vi "Top_Level_Control_1SDI_v00.vi"() -> ()   [LabVIEW 2011]
uses:
  Strict Type Defs/Control GUI 1SDI HD.ctl
  Strict Type Defs/PII Gains.ctl
  Strict Type Defs/I16 white control.ctl
  Strict Type Defs/Thresh slider.ctl
  Strict Type Defs/Lock or Hold.ctl
  Strict Type Defs/Scan Freq Slider.ctl
  Strict Type Defs/Gains negative horizontal.ctl
  Strict Type Defs/Slider and display.ctl
  Strict Type Defs/theta 1SDI.ctl
  Strict Type Defs/Control GUI 1SDI EPR.ctl
  Strict Type Defs/Lock Select 1SDI.ctl
  Strict Type Defs/Scope and Safety.ctl
  Strict Type Defs/Hold All.ctl
  <vilib>/userdefined/High Color/nirio_resource_hc.ctl
  Strict Type Defs/Extras 1SDI.ctl
  Strict Type Defs/Double ISDI control.ctl
  Strict Type Defs/I16 1SDI Control.ctl
  <vilib>/FPGAPlugInAG/PXI-7852R/niLvFpga_Open_PXI-7852R.vi
  <vilib>/rvi/interface/common/dynamic/niFpgaDynamicAddResources.vi
  <vilib>/Utility/error.llb/Error Cluster From Error Code.vi
  <vilib>/rvi/errors/niLvFpgaAdjustHostInterfaceError.vi
  <vilib>/FPGAPlugInAG/Dynamic/niLvFpga_Close_Dynamic.vi
  <vilib>/rvi/interface/nirviOpenFPGA/nirviOpenFPGA.xnode
  FPGA Bitfiles/1SDI_FPGATarget_1SDIFPGAv00_0D511EDE.lvbitx
  <vilib>/rvi/interface/nirviReadWriteControl/nirviReadWriteControl.xnode
  <vilib>/rvi/interface/nirviMethod/nirviMethod.xnode
  <vilib>/rvi/interface/nirviCloseFPGA/nirviCloseFPGA.xnode
  <vilib>/FPGAPlugInAG/Dynamic/niLvFpga_ReadFifo_Dynamic.vi
  <vilib>/rvi/errors/niLvFpgaMergeErrorWithErrorCode.vi
  NiFpgaLv.dll
  <vilib>/rvi/interface/Simulation/niFpgaSimulationCallBeginRW.vi
panel:
  in  "watertank":bool
  out "Water Tank":dbl(slide)=-0.29411764705882354 scale=-0.3..0.3
  out "Top Loop Count":i32=272090
  in  "stop":bool
  in  "Hold All":T1
  in  "Extra Controls":enum32{"Scope", "Extra Controls", "X-Y Resurge"}(tab)
  in  "Scope+Safety":T2={"Safety First"={"lim reset"=FALSE, "no limit"=FALSE, "pos slew rate * dt"=12, "neg slew rate * dt"=-12, "Count(Ticks)"=0}, "Scope IPs"={"Trigger Direction"=enum."minus-plus", "Trigger Delay (ms)"=0.0, "Aquisition Rate (kHz)"=4000.0, "Trigger Offset (V)"=0.0, "Scale Offset"={"Scaling"={"Error signal"=1, "Output"=0, "DC Monitor"=1, "Threshold"=1}, "Offset"={"Error Signal"=0, "Output"=0, "DC Monitor"=0, "Threshold"=0}}}}
  in  "Extras 1SDI":T3={"Error Bit Shift "={"EPR BS"=0, "HD A x"=0, "HD A p"=0, "HD B x"=0, "HD B p"=0}, "I Max value"=20000, "Scan Offset"={"EPR BS"=0.0, "HD A"=0.0, "HD B"=0.0}, "Scan Ampl."={"EPR BS"=0.0, "HD A"=0.0, "HD B"=0.0}, "Scan-PII thresh"={"EPR BS"=0, "Homodyne A"=0, "Homodyne B"=0}, "Re-Scan thresh"={"EPR BS"=1000, "Homodyne A"=1000, "Homodyne B"=1000}, "Post-Offset"={"HD A x"=0.0, "HD A p"=0.0, "HD B x"=0.0, "HD B p"=0.0}}
  out "Graph error":errorcluster
  in  "Number of Elements":u32=4095
  in  "1SDI_FPGA_v00":T6="RIO1" caption="RIO Device"
  out "xy HD A":cluster{i16[], i16[]}(graph)
  in  "XY HD ON":bool
  out "xy HD B":cluster{i16[], i16[]}(graph)
  in  "Scope":T7=TRUE
  out "Scope Graph":cluster{dbl[], dbl[]}[](graph)
  in  "Lock Select":T8=enum."Homodyne B"
  in  "EPR BS":T9={"Offset Error"=-0.0003333333333333334, "Gain Error"=1, "P Gain"=25, "P Bit Shift"=-10, "I Bit Shift"=-10, "I Gain"=23, "Lock Threshold"=22, "Lock"=FALSE, "Hold"=FALSE, "Scan Frequency"=17, "Scan Bit Shift"=-4, "Gains +/- "=FALSE, "Pre- Offset Error"=0.0005084745762711861} {"Pre- Offset Error" scale=-0.01..0.01 scale format="%#_5f"; "Scan Frequency" scale=1.0..30.0; "I Gain" scale=0.0..50.0; "P Gain" scale=0.0..50.0; "Offset Error" scale=-0.01..0.01 scale format="%#_5f"}
  in  "Homodyne A":T16={"P Gain"=27, "P Bit Shift"=-8, "I Bit Shift"=-8, "I Gain"=19, "Lock Threshold"=37, "Lock"=FALSE, "Hold"=FALSE, "Scan Frequency"=13, "Scan Bit Shift"=-5, "Gains +/- "=FALSE, "Pre- Offset x"=0.0008474576271186437, "Pre-Offset p"=-0.0023163841807909607, "Gain Error x"=1, "Lock Angle"=0.0, "Gain Error p\n\n"=1} {"Lock Angle" min=-90.0 max=90.0 scale=-90.0..90.0 scale format="%#_2g"; "Pre-Offset p" scale=-0.01..0.01 scale format="%#_5f"; "Pre- Offset x" scale=-0.01..0.01 scale format="%#_5f"; "Scan Frequency" scale=1.0..30.0; "I Gain" scale=0.0..50.0; "P Gain" scale=0.0..50.0}
  in  "Homodyne B":T16={"P Gain"=14, "P Bit Shift"=-8, "I Bit Shift"=-8, "I Gain"=22, "Lock Threshold"=48, "Lock"=FALSE, "Hold"=FALSE, "Scan Frequency"=19, "Scan Bit Shift"=-5, "Gains +/- "=FALSE, "Pre- Offset x"=-0.0016384180790960455, "Pre-Offset p"=-0.002090395480225989, "Gain Error x"=1, "Lock Angle"=15.0, "Gain Error p\n\n"=1} {"Lock Angle" min=-90.0 max=90.0 scale=-90.0..90.0 scale format="%#_2g"; "Pre-Offset p" scale=-0.01..0.01 scale format="%#_5f"; "Pre- Offset x" scale=-0.01..0.01 scale format="%#_5f"; "Scan Frequency" scale=1.0..30.0; "I Gain" scale=0.0..50.0; "P Gain" scale=0.0..50.0}
  # "Error Signal"
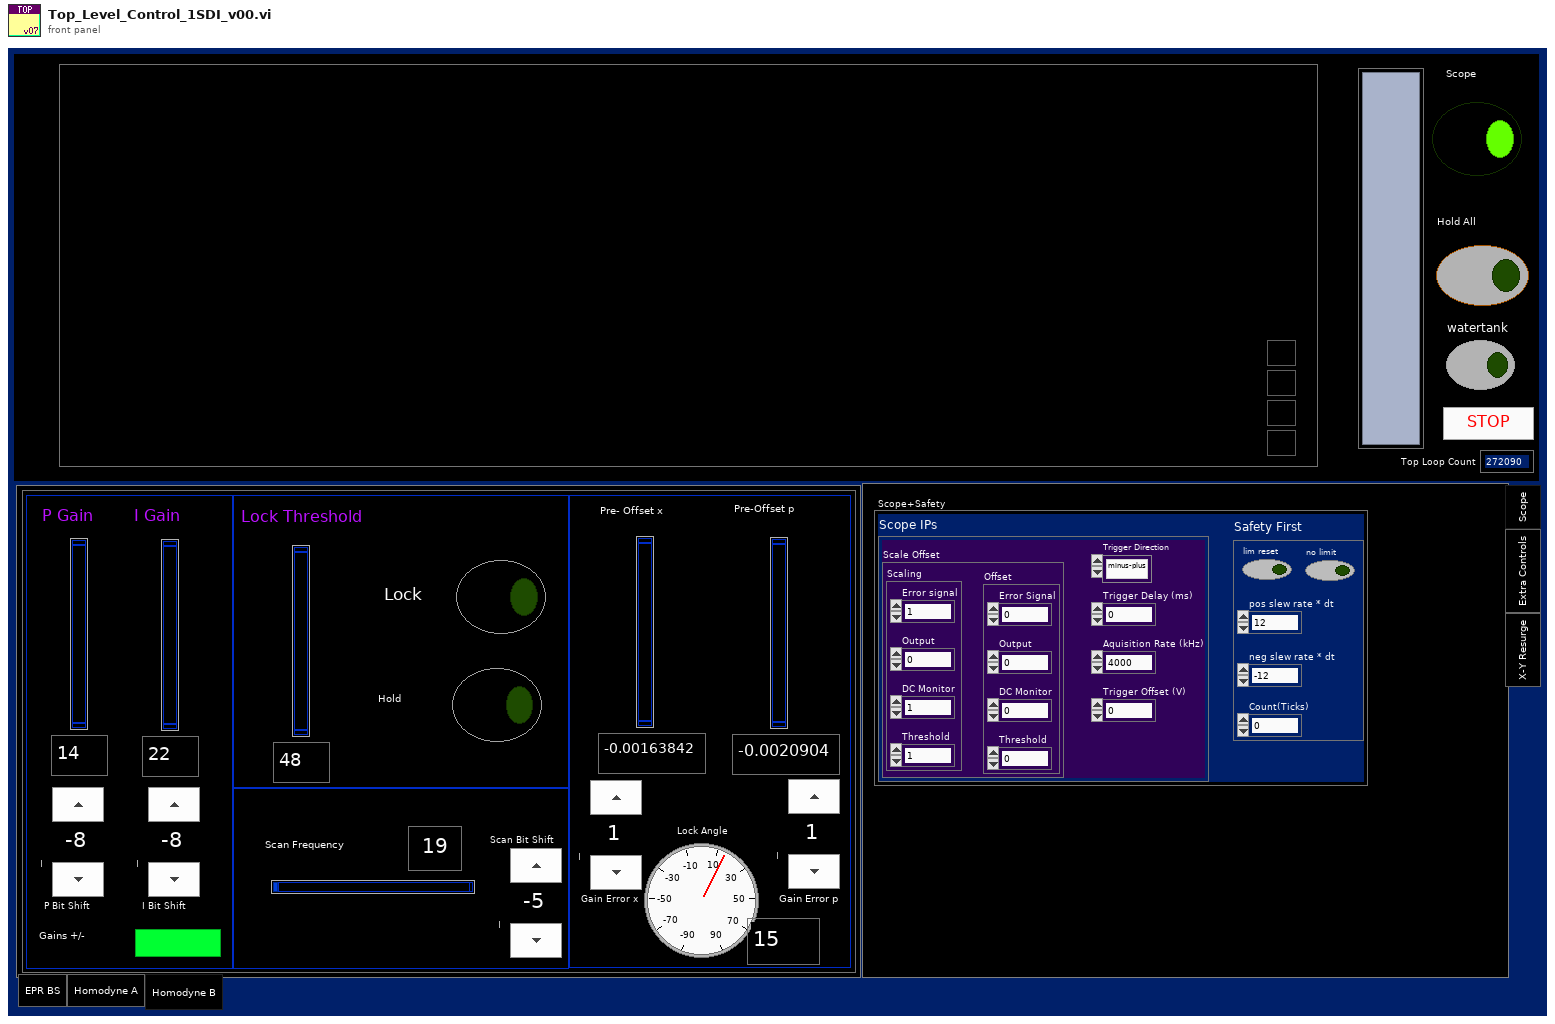
[diagram p1: front panel]
types:
  T1 = typedef "Hold All.ctl" = bool
  T2 = typedef "Scope and Safety.ctl" = cluster{"Safety First":cluster{"lim reset":bool, "no limit":bool, "pos slew rate * dt":i16, "neg slew rate * dt":i16, "Count(Ticks)":u32}, "Scope IPs":cluster{"Trigger Direction":enum8{"either", "minus-plus", "plus-minus"}, "Trigger Delay (ms)":dbl, "Aquisition Rate (kHz)":dbl, "Trigger Offset (V)":dbl, "Scale Offset":cluster{"Scaling":cluster{"Error signal":i16, "Output":i16, "DC Monitor":i16, "Threshold":i16}, "Offset":cluster{"Error Signal":i16, "Output":i16, "DC Monitor":i16, "Threshold":i16}}}}
  T3 = typedef "Extras 1SDI.ctl" = cluster{"Error Bit Shift ":cluster{"EPR BS":i16, "HD A x":i16, "HD A p":i16, "HD B x":i16, "HD B p":i16}, "I Max value":i32, "Scan Offset":T4, "Scan Ampl.":T4, "Scan-PII thresh":T5, "Re-Scan thresh":T5, "Post-Offset":cluster{"HD A x":dbl, "HD A p":dbl, "HD B x":dbl, "HD B p":dbl}}
  T4 = typedef "Double ISDI control.ctl" = cluster{"EPR BS":dbl, "HD A":dbl, "HD B":dbl}
  T5 = typedef "I16 1SDI Control.ctl" = cluster{"EPR BS":i16, "Homodyne A":i16, "Homodyne B":i16}
  T6 = typedef "nirio_resource_hc.ctl" = tag
  T7 = typedef "Lock or Hold.ctl" = bool
  T8 = typedef "Lock Select 1SDI.ctl" = enum32{"EPR BS", "Homodyne A", "Homodyne B"}
  T9 = typedef "Control GUI 1SDI EPR.ctl" = cluster{"Offset Error":T10, "Gain Error":T11, "P Gain":T12, "P Bit Shift":T11, "I Bit Shift":T11, "I Gain":T12, "Lock Threshold":T13, "Lock":T7, "Hold":T7, "Scan Frequency":T14, "Scan Bit Shift":T11, "Gains +/- ":T15, "Pre- Offset Error":T10}
  T10 = typedef "Slider and display.ctl" = dbl
  T11 = typedef "I16 white control.ctl" = i16
  T12 = typedef "PII Gains.ctl" = i32
  T13 = typedef "Thresh slider.ctl" = i16
  T14 = typedef "Scan Freq Slider.ctl" = u16
  T15 = typedef "Gains negative horizontal.ctl" = bool
  T16 = typedef "Control GUI 1SDI HD.ctl" = cluster{"P Gain":T12, "P Bit Shift":T11, "I Bit Shift":T11, "I Gain":T12, "Lock Threshold":T13, "Lock":T7, "Hold":T7, "Scan Frequency":T14, "Scan Bit Shift":T11, "Gains +/- ":T15, "Pre- Offset x":T10, "Pre-Offset p":T10, "Gain Error x":T11, "Lock Angle":T17, "Gain Error p\n\n":T11}
  T17 = typedef "theta 1SDI.ctl" = dbl
  T18 = cluster{"PII In 1":cluster{"Lock":bool, "Hold":bool, "P Gain":i32, "P BS":i16, "I Gain":i32, "I BS":i16, "I2 G":i32, "I2 BS":i16, "Scan Amp":i16, "Scan Off":i16, "Scan FS":u16, "SFS BS":i16, "I Max value":i32, "I2 Max value":i32, "Scope.Offset":i16, "Trigger Direction":enum8{"either", "minus-plus", "plus-minus"}, "Scan-PII thresh":i16}, "PII In 2":cluster{"Lock":bool, "Hold":bool, "P Gain":i32, "P BS":i16, "I Gain":i32, "I BS":i16, "I2 G":i32, "I2 BS":i16, "Scan Amp":i16, "Scan Off":i16, "Scan FS":u16, "SFS BS":i16, "I Max value":i32, "I2 Max value":i32, "Scope.Offset":i16, "Trigger Direction":enum8{"either", "minus-plus", "plus-minus"}, "Scan-PII thresh":i16}, "PII In 3":cluster{"Lock":bool, "Hold":bool, "P Gain":i32, "P BS":i16, "I Gain":i32, "I BS":i16, "I2 G":i32, "I2 BS":i16, "Scan Amp":i16, "Scan Off":i16, "Scan FS":u16, "SFS BS":i16, "I Max value":i32, "I2 Max value":i32, "Scope.Offset":i16, "Trigger Direction":enum8{"either", "minus-plus", "plus-minus"}, "Scan-PII thresh":i16}, "Error scale":cluster{"Pre-Offset":cluster{"Pre-Offset 1":i16, "Pre-Offset 2":i16, "Pre-Offset 3":i16, "Pre-Offset 4":i16, "Pre-Offset 5":i16}, "Post-Offset ":cluster{"Offset 1":i16, "Offset 2":i16, "Offset 3":i16, "Offset 4":i16, "Offset 5":i16}, "Gains":cluster{"Gain 1":i16, "Gain 2":i16, "Gain 3":i16, "Gain 4":i16, "Gain 5":i16}, "Bit Shifts":cluster{"Bit Shift 1":i16, "Bit Shift 2":i16, "Bit Shift 3":i16, "Bit Shift 4":i16, "Bit Shift 5":i16}}, "Lock Thresh":cluster{"EPR":i16, "HD A":i16, "HD B":i16}, "Re-Scan Thresh":cluster{"EPR":i16, "HD A":i16, "HD B":i16}, "Theta":cluster{"HD A Sin Theta":i32, "HD A Cos Theta":i32, "HD B Sin Theta":i32, "HD B Cos Theta":i32}, "Safety First":cluster{"lim reset":bool, "no limit":bool, "pos slew rate * dt":i16, "neg slew rate * dt":i16, "Hold All":bool, "Count(Ticks)":u32}}
  T19 = cluster{"Trigger Direction":enum8{"either", "minus-plus", "plus-minus"}, "Delay":u32, "Aquisition Rate (Ticks)":u32, "Offset":i16, "Channel":i32, "Channel Selector":cluster{"Channel 1":i32, "Channel 2":i32, "Channel 3":i32, "Channel 4":i32}}
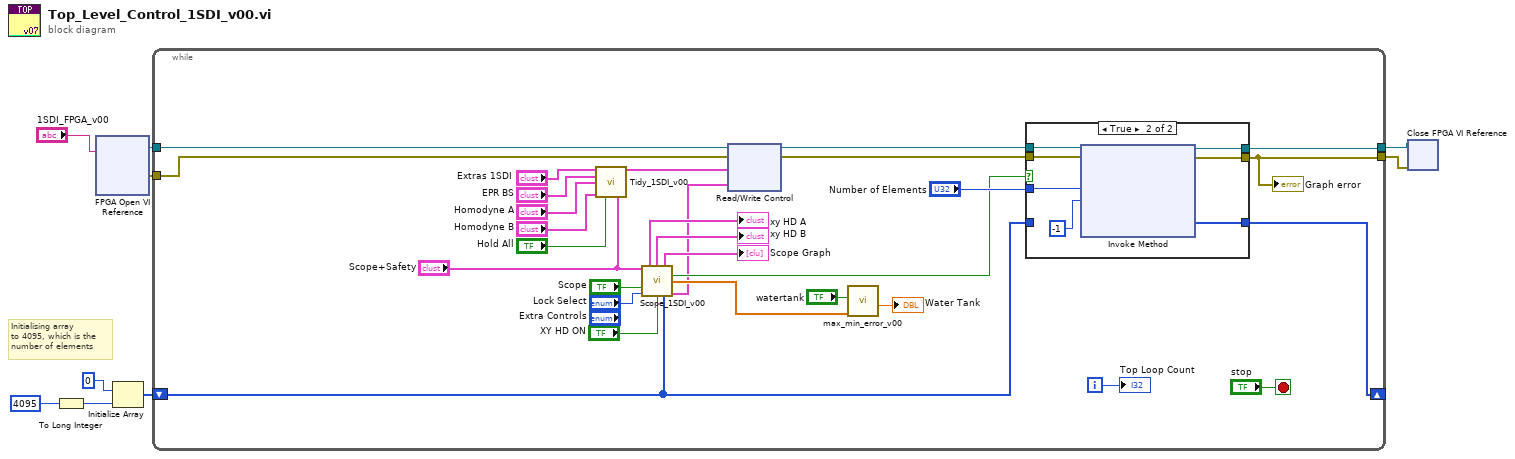
[diagram p0: block diagram]
diagram:
  # "Initialising array\nto 4095, which is the\nnumber of elements"
  n1 = To Long Integer(number=4095) -> (32bit integer=w9:i32)
  n2 = xnode "FPGA Open VI Reference"("resource name"="1SDI_FPGA_v00") -> ("FPGA VI Reference Out"=w5:refnum<k20>, "error out"=w4:errorcluster)  [unwired: 1 in]
  n3 = Initialize Array(u64 0 ("element"), w9) -> (w1:u64[])
  n4 = while {
    tunnel: w5 -> [w21]
    tunnel: w4 -> [w20]
    tunnel: [w35] -> w3
    tunnel: [w34] -> w2
    shift-right: [w32] -> _
    shift-left: w1 -> [w31]
    i -> [w37]
    stop <- "stop" stop-if-true
    n5 = call "Tidy_1SDI_v00.vi"("Extras 1SDI"="Extras 1SDI", "EPR BS"="EPR BS", "Homodyne A"="Homodyne A", "Homodyne B"="Homodyne B", "Hold All"="Hold All", "Scope+Safety"="Scope+Safety") -> ("1SDI Control"=w13:T18)  [unwired: 9 in]
    n6 = call "Scope_1SDI_v00.vi"("Scope+Safety"="Scope+Safety", "Scope"="Scope", "Lock Select"="Lock Select", "XY HD ON"="XY HD ON", "1SDI Data"=w31) -> ("xy HD A"=→"xy HD A":cluster{i16[], i16[]}, "xy HD B"=→"xy HD B":cluster{i16[], i16[]}, "Scope OP 1SDI"=→"Scope Graph":cluster{dbl[], dbl[]}[], "Scope 1SDI ON"=w28:bool, "error"=w24:dbl[], "Scope 1SDI FPGA"=w12:T19)  [unwired: 5 in]
    n7 = xnode "Read/Write Control"("FPGA VI Reference In"=w21, "error in"=w20, "Control"=w13, "Scope"=w12) -> ("FPGA VI Reference Out"=w19:refnum<k20>, "error out"=w18:errorcluster)
    n8 = call "max_min_error_v00.vi"("Array"=w24, "maxmin"="watertank") -> ("x+y"=→"Water Tank":dbl)  [unwired: 7 in, 2 out]
    n9 = case shown="True" w28 {
      tunnel: w18 -> [w41 w48]
      tunnel: [w41 w47] -> w34
      tunnel: w19 -> [w40 w46]
      tunnel: [w40 w45] -> w35
      tunnel: [w39 w44] -> w32
      tunnel: w31 -> [w39 _]
      tunnel: "Number of Elements" -> [_ w42]
      frame False {
      }
      frame True {
        n10 = xnode "Invoke Method"("FPGA VI Reference In"=w46, "error in"=w48, "Number of Elements"=w42, "Timeout (ms)"=-1) -> ("FPGA VI Reference Out"=w45:refnum<k20>, "error out"=w47:errorcluster, "Data"=w44:u64[])  [unwired: 1 out]
      }
    }
    "Graph error" <- w34
    "Top Loop Count" <- w37
  }
  n11 = xnode "Close FPGA VI Reference"("FPGA VI Reference In"=w3, "error in"=w2) -> ()  [unwired: 1 out]
